vi "Configure Crop New.vi"(6 "Codec":string, 7 "State In":T1, 8 "error in (no error)":errorcluster, 9 "Time Crop Method":T3, 10 "Annotation List":T2[](array[typedef]) {"Frame Start" min=0}, 11 "Frame Grabber Data In":T4={"Camera Session"="", "Frame"=refnum, "AVI Refnum"=refnum, "Codecs"=[], "Frame number"=0, "Tracking File Refnum"=refnum, "Tick Count"=0, "Probe Object"=refnum, "Playback Probe Data"=[], "Rigid Body"={"Position"={"x (mm)"=0.0, "y (mm)"=0.0, "z (mm)"=0.0}, "Orientation"={"Pitch (rad)"=0.0, "Yaw (rad)"=0.0, "Roll (rad)"=0.0}, "Quaternion"={"qx"=0.0, "qy"=0.0, "qz"=0.0, "qw"=0.0}, "Tracked?"=FALSE}, "Total no frames playback"=0, "Video FPS"=0.0, "Camera connected?"=FALSE, "Scene"=refnum, "Cropped Frame"=refnum, "Tracker FPS"=0.0, "Crop ROI"=[], "Presentation Values"=[], "Elapsed time (ms)"=0, "Camera frames playback"=0, "Refnums"={"Live Refnum"=refnum, "Record Refnum"=refnum, "Playback Refnum"=refnum, "Frame Slider Refnum"=refnum, "Pause Refnum"=refnum, "Home Refnum"=refnum, "Set Crop Refnum"=refnum, "Clear Crop Refnum"=refnum, "stop refnum"=refnum, "Playback Rate Refnum"=refnum, "Presentation Refnum"=refnum, "Crop Time Frame Slider Refnum"=refnum, "Cancel Save Refnum"=refnum, "Reverse Playback Refnum"=refnum, "Recording Settings Refnum"=refnum, "Continuous Playback Refnum"=refnum, "Annotation Refnum"=refnum, "Export All Refnum"=refnum, "Export List Refnum"=refnum, "Fill List Refnum"=refnum, "Save Crop Refnum"=refnum, "Skip Forward Refnum"=refnum, "Skip Backward Refnum"=refnum, "Single Annotation Refnum"=refnum, "Load Refnum"=refnum, "Set Start Refnum"=refnum, "Set End Refnum"=refnum, "Add to List Refnum"=refnum, "List of Annotations Refnum"=refnum, "Camera Frame Refnum"=refnum}, "Dimensions"={"Probe Dimensions"={"Probe Width"=0.0, "Probe Depth"=1.0, "Probe Height"=0.0}, "Room Dimensions"={"Room Width"=0.0, "Room Depth"=0.0, "Room Height"=0.0}}, "Playback Data As Strings"=[], "Cropped Tracking File Refnum"=refnum, "Cropped AVI Refnum"=refnum, "Header"=[], "Total euclidian distance"=0.0, "Annotation File Path"=path "", "Playback File Path"=path "", "Size per frame"=0.0, "Ground Truth File Refnum"=refnum, "Annotation Array"=[], "Annotation TIFFs Folder"=path "", "overwriting open file?"=FALSE}) -> (0 "error out":errorcluster, 1 "Valid crop region?":bool, 2 "Saving?":bool, 3 "Frame Grabber Data Out":T4={"Camera Session"="", "Frame"=refnum, "AVI Refnum"=refnum, "Codecs"=[], "Frame number"=0, "Tracking File Refnum"=refnum, "Tick Count"=0, "Probe Object"=refnum, "Playback Probe Data"=[], "Rigid Body"={"Position"={"x (mm)"=0.0, "y (mm)"=0.0, "z (mm)"=0.0}, "Orientation"={"Pitch (rad)"=0.0, "Yaw (rad)"=0.0, "Roll (rad)"=0.0}, "Quaternion"={"qx"=0.0, "qy"=0.0, "qz"=0.0, "qw"=0.0}, "Tracked?"=FALSE}, "Total no frames playback"=0, "Video FPS"=0.0, "Camera connected?"=FALSE, "Scene"=refnum, "Cropped Frame"=refnum, "Tracker FPS"=0.0, "Crop ROI"=[], "Presentation Values"=[], "Elapsed time (ms)"=0, "Camera frames playback"=0, "Refnums"={"Live Refnum"=refnum, "Record Refnum"=refnum, "Playback Refnum"=refnum, "Frame Slider Refnum"=refnum, "Pause Refnum"=refnum, "Home Refnum"=refnum, "Set Crop Refnum"=refnum, "Clear Crop Refnum"=refnum, "stop refnum"=refnum, "Playback Rate Refnum"=refnum, "Presentation Refnum"=refnum, "Crop Time Frame Slider Refnum"=refnum, "Cancel Save Refnum"=refnum, "Reverse Playback Refnum"=refnum, "Recording Settings Refnum"=refnum, "Continuous Playback Refnum"=refnum, "Annotation Refnum"=refnum, "Export All Refnum"=refnum, "Export List Refnum"=refnum, "Fill List Refnum"=refnum, "Save Crop Refnum"=refnum, "Skip Forward Refnum"=refnum, "Skip Backward Refnum"=refnum, "Single Annotation Refnum"=refnum, "Load Refnum"=refnum, "Set Start Refnum"=refnum, "Set End Refnum"=refnum, "Add to List Refnum"=refnum, "List of Annotations Refnum"=refnum, "Camera Frame Refnum"=refnum}, "Dimensions"={"Probe Dimensions"={"Probe Width"=0.0, "Probe Depth"=1.0, "Probe Height"=0.0}, "Room Dimensions"={"Room Width"=0.0, "Room Depth"=0.0, "Room Height"=0.0}}, "Playback Data As Strings"=[], "Cropped Tracking File Refnum"=refnum, "Cropped AVI Refnum"=refnum, "Header"=[], "Total euclidian distance"=0.0, "Annotation File Path"=path "", "Playback File Path"=path "", "Size per frame"=0.0, "Ground Truth File Refnum"=refnum, "Annotation Array"=[], "Annotation TIFFs Folder"=path "", "overwriting open file?"=FALSE}, 5 "State Out":T1=enum."Multi-Crop")   [LabVIEW 2017]
uses:
  Controls/Frame Grabber Data.ctl
  <vilib>/userdefined/High Color/IMAQdx.ctl
  <vilib>/vision/Image Controls.llb/IMAQ Image.ctl
  <vilib>/vision/Avi.llb/IMAQ AVI2 Refnum.ctl
  Controls/Rigid Body Info.ctl
  Controls/Position.ctl
  Controls/Orientation.ctl
  Controls/Refnums.ctl
  Controls/Recording Settings.ctl
  Controls/Operator Settings.ctl
  Controls/Operator.ctl
  Controls/Patient Settings.ctl
  Controls/Dimensions.ctl
  Controls/Room Dimensions.ctl
  Controls/Time Crop Method.ctl
  Controls/Annotation Sequence Details.ctl
  Controls/Crop Video State.ctl
panel:
  out "Playback File Path":path
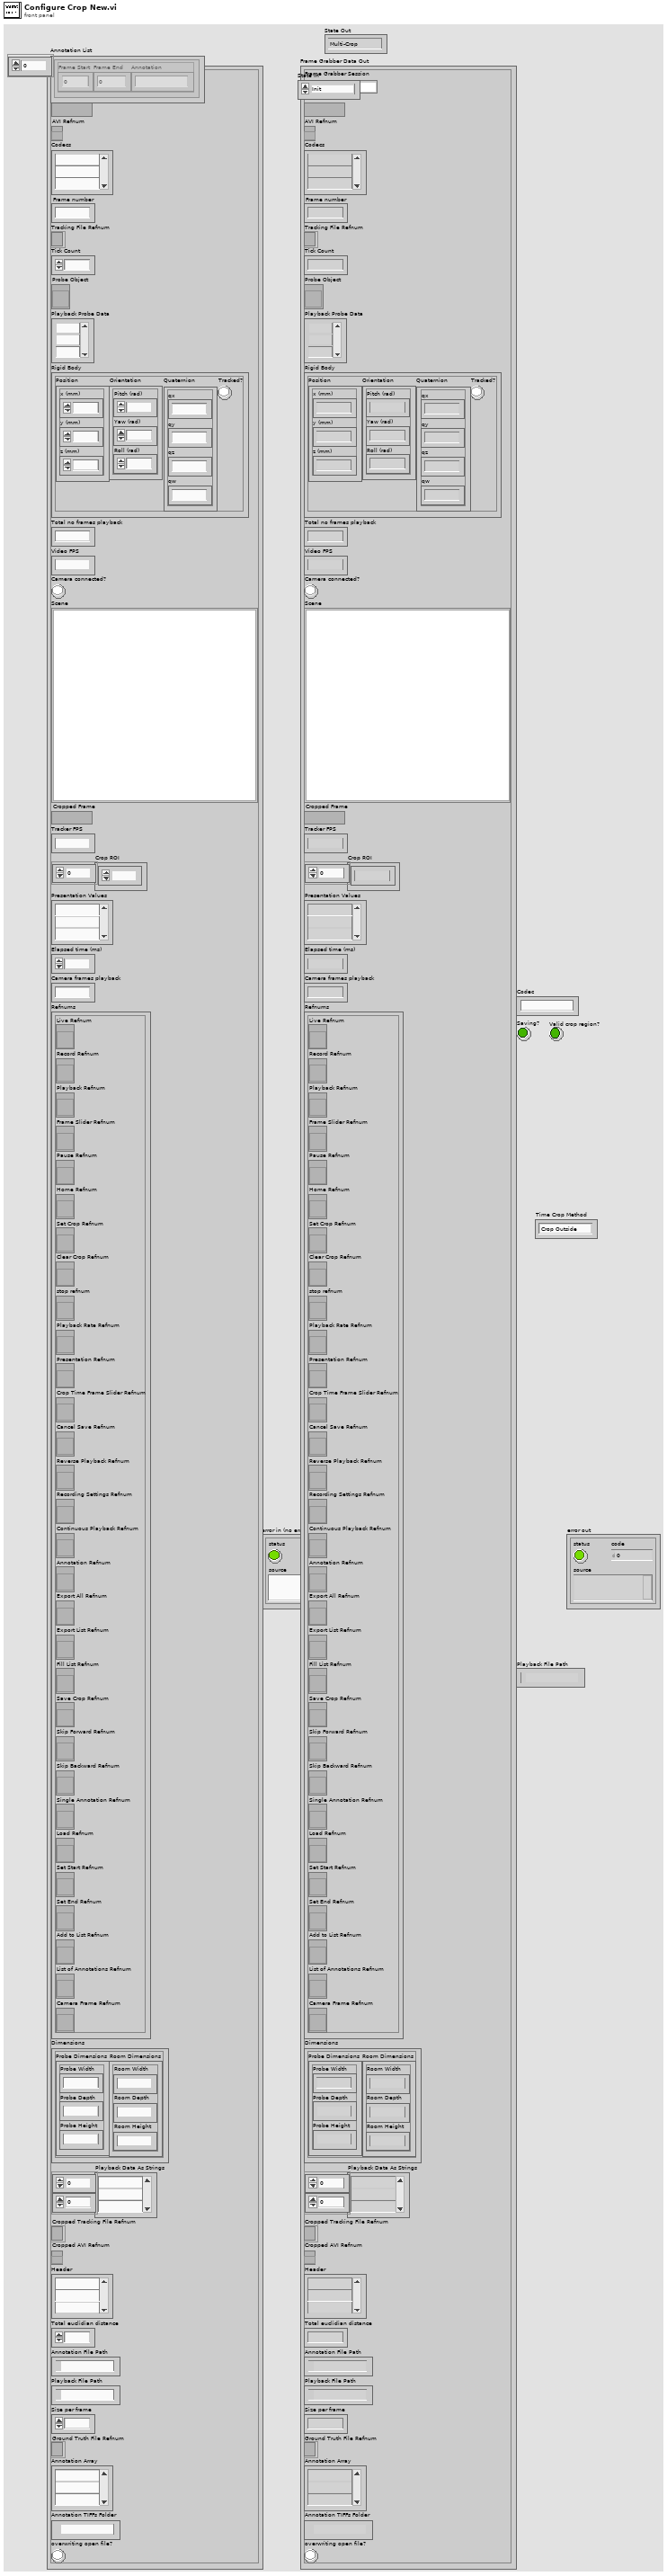
[diagram p1: front panel]
types:
  T1 = typedef "Crop Video State.ctl" = enum16{"Init", "Wait", "Load", "Playback Frame", "Save", "Export List", "Export All", "Close", "Set Crop Area", "Reset Crop Area", "Crop Inside", "Crop Outside", "Multi-Crop", "Re-Open Files", "Annotate Frame", "Annotate Clip", "Add to List", "Fill List", "Set Start", "Set End", "Error Handling", "Shutdown"}
  T2 = typedef "Annotation Sequence Details.ctl" = cluster{"Frame Start":i32, "Frame End":i32, "Annotation":string}
  T3 = typedef "Time Crop Method.ctl" = enum16{"Crop Outside", "Crop Inside"}
  T4 = typedef "Frame Grabber Data.ctl" = cluster{"Camera Session":T5, "Frame":T6, "AVI Refnum":T7, "Codecs":string[], "Frame number":u32, "Tracking File Refnum":refnum<file>, "Tick Count":u32, "Probe Object":refnum<vi>, "Playback Probe Data":dbl[][], "Rigid Body":T8, "Total no frames playback":i32, "Video FPS":dbl, "Camera connected?":bool, "Scene":refnum<vi>, "Cropped Frame":T6, "Tracker FPS":dbl, "Crop ROI":i32[], "Presentation Values":string[], "Elapsed time (ms)":u32, "Camera frames playback":u32, "Refnums":T11, "Dimensions":T12, "Playback Data As Strings":string[][], "Cropped Tracking File Refnum":refnum<file>, "Cropped AVI Refnum":T7, "Header":string[], "Total euclidian distance":dbl, "Annotation File Path":path, "Playback File Path":path, "Size per frame":dbl, "Ground Truth File Refnum":refnum<file>, "Annotation Array":string[], "Annotation TIFFs Folder":path, "overwriting open file?":bool}
  T5 = typedef "IMAQdx.ctl" = refnum<k21>
  T6 = typedef "IMAQ Image.ctl" = refnum<image>
  T7 = typedef "IMAQ AVI2 Refnum.ctl" = refnum<k20>
  T8 = typedef "Rigid Body Info.ctl" = cluster{"Position":T9, "Orientation":T10, "Quaternion":cluster{"qx":sgl, "qy":sgl, "qz":sgl, "qw":sgl}, "Tracked?":bool}
  T9 = typedef "Position.ctl" = cluster{"x (mm)":sgl, "y (mm)":sgl, "z (mm)":sgl}
  T10 = typedef "Orientation.ctl" = cluster{"Pitch (rad)":sgl, "Yaw (rad)":sgl, "Roll (rad)":sgl}
  T11 = typedef "Refnums.ctl" = cluster{"Live Refnum":refnum<vi>, "Record Refnum":refnum<vi>, "Playback Refnum":refnum<vi>, "Frame Slider Refnum":refnum<vi>, "Pause Refnum":refnum<vi>, "Home Refnum":refnum<vi>, "Set Crop Refnum":refnum<vi>, "Clear Crop Refnum":refnum<vi>, "stop refnum":refnum<vi>, "Playback Rate Refnum":refnum<vi>, "Presentation Refnum":refnum<vi>, "Crop Time Frame Slider Refnum":refnum<vi>, "Cancel Save Refnum":refnum<vi>, "Reverse Playback Refnum":refnum<vi>, "Recording Settings Refnum":refnum<vi>, "Continuous Playback Refnum":refnum<vi>, "Annotation Refnum":refnum<vi>, "Export All Refnum":refnum<vi>, "Export List Refnum":refnum<vi>, "Fill List Refnum":refnum<vi>, "Save Crop Refnum":refnum<vi>, "Skip Forward Refnum":refnum<vi>, "Skip Backward Refnum":refnum<vi>, "Single Annotation Refnum":refnum<vi>, "Load Refnum":refnum<vi>, "Set Start Refnum":refnum<vi>, "Set End Refnum":refnum<vi>, "Add to List Refnum":refnum<vi>, "List of Annotations Refnum":refnum<vi>, "Camera Frame Refnum":refnum<vi>}
  T12 = typedef "Dimensions.ctl" = cluster{"Probe Dimensions":cluster{"Probe Width":sgl, "Probe Depth":sgl, "Probe Height":sgl}, "Room Dimensions":T13}
  T13 = typedef "Room Dimensions.ctl" = cluster{"Room Width":dbl, "Room Depth":dbl, "Room Height":dbl}
  T14 = enum16{"open", "replace", "create", "open or create", "replace or create", "replace or create with confirmation"}
  T15 = cluster{"Width":u32, "Height":u32, "Frames Per Second":u32, "Codec":string, "Has Data":bool}
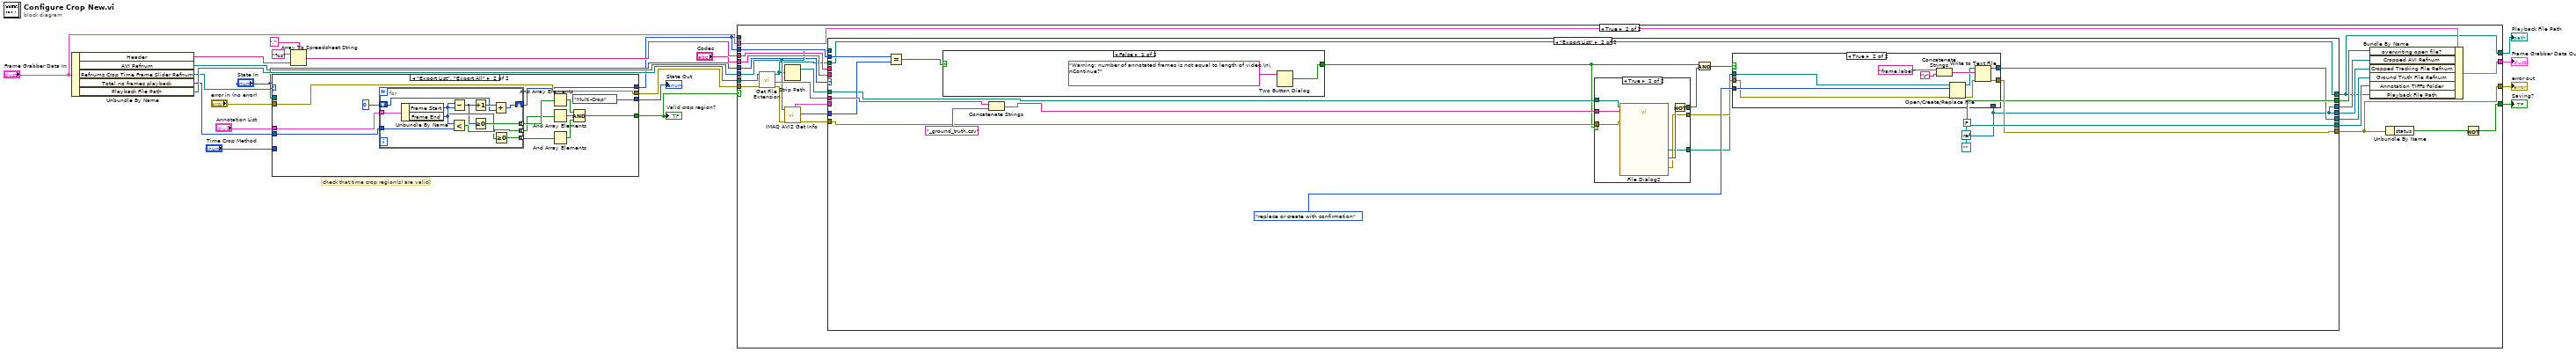
[diagram p0: block diagram]
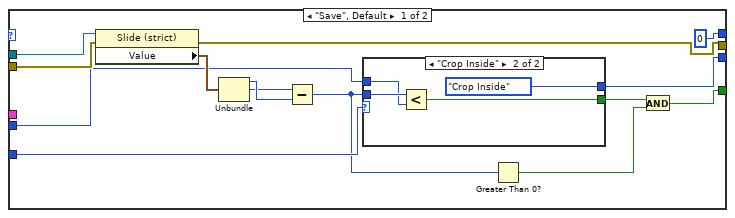
[diagram p2: hidden frame]
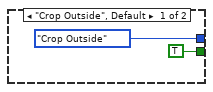
[diagram p3: hidden frame]
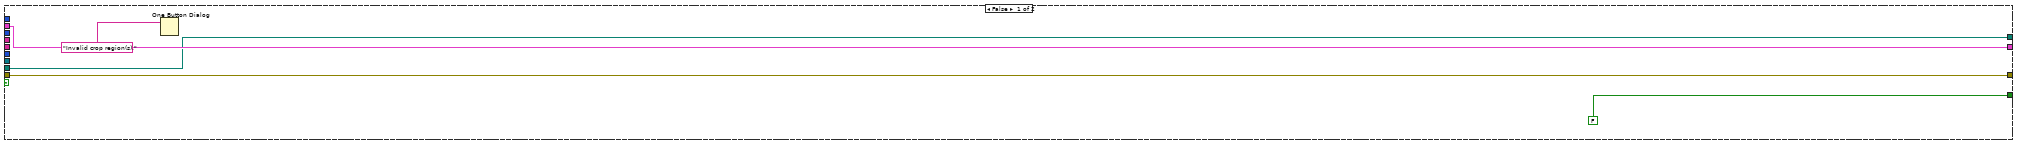
[diagram p4: hidden frame]
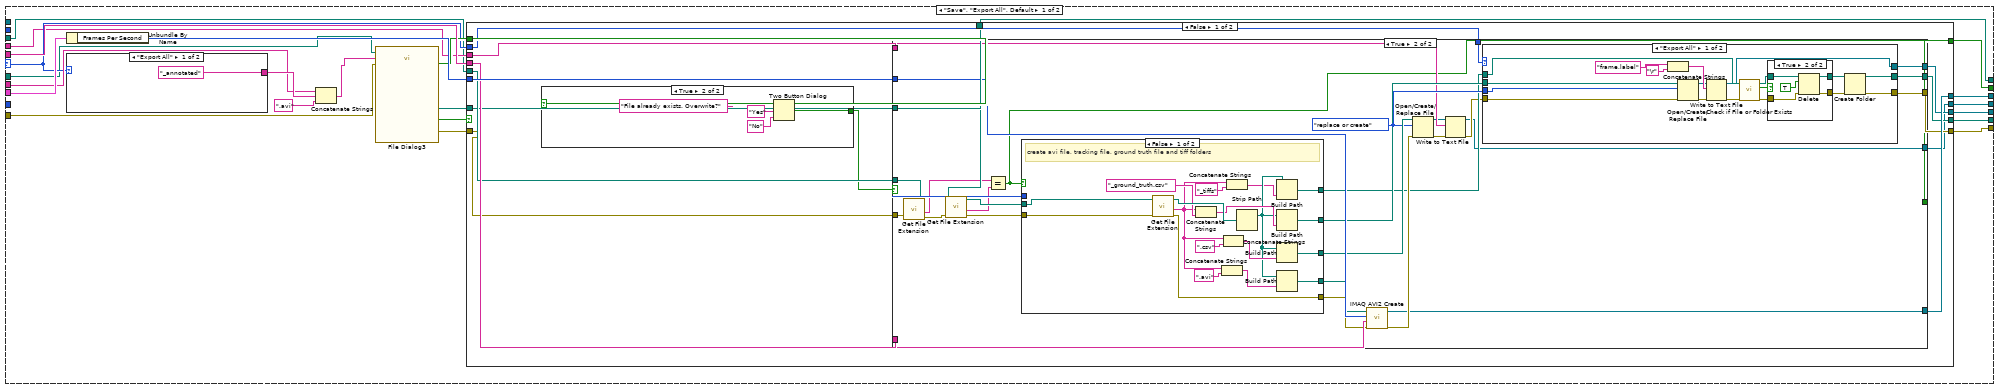
[diagram p5: hidden frame]
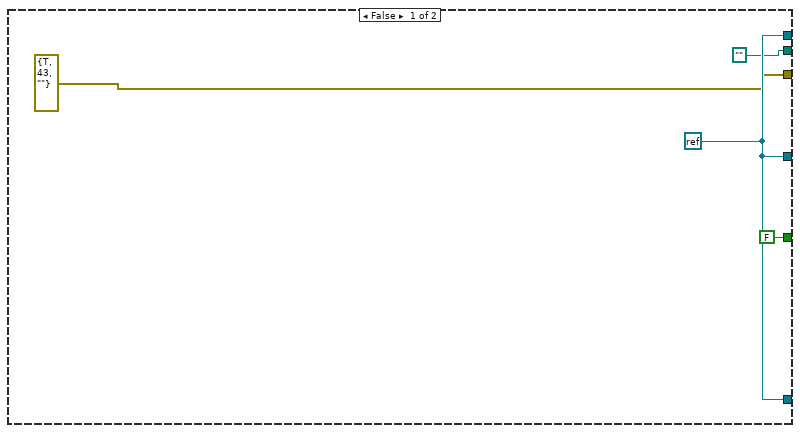
[diagram p6: hidden frame]
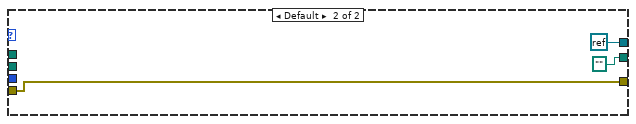
[diagram p8: hidden frame]
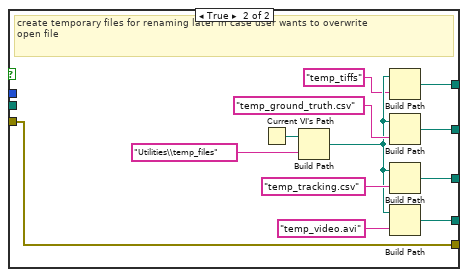
[diagram p9: hidden frame]
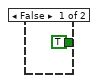
[diagram p10: hidden frame]
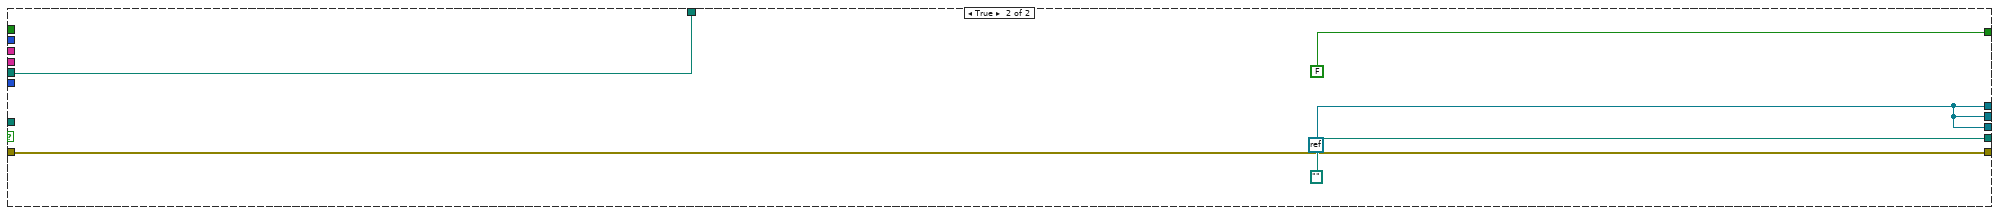
[diagram p11: hidden frame]
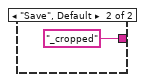
[diagram p12: hidden frame]
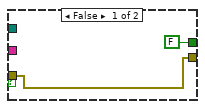
[diagram p13: hidden frame]
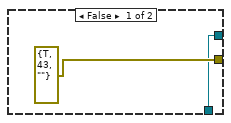
[diagram p14: hidden frame]
diagram:
  # "check that time crop region(s) are valid!"
  n1 = Unbundle By Name("Frame Grabber Data In") -> ("Header"=w16:string[], "AVI Refnum"=w3:T7, "Refnums.Crop Time Frame Slider Refnum"=w13:refnum<vi>, "Total no frames playback"=w9:i32, "Playback File Path"=w17:path)
  n2 = case shown="\"Export List\", \"Export All\"" "State In" {
    tunnel: "Annotation List" -> [_ w55]
    tunnel: w13 -> [w33 _]
    tunnel: "error in (no error)" -> [w32 w53]
    tunnel: [w31 w53] -> w11
    tunnel: "Time Crop Method" -> [w30 _]
    tunnel: w9 -> [w29 w51]
    tunnel: [w25 w46] -> w8
    tunnel: [w24 Crop_Video_State."Multi-Crop" ("State")] -> w7
    tunnel: [0 w43] -> w2
    frame "Save", Default {
      n3 = property class="Slide (strict)"(reference=w33, error in=w32) -> (error out=w31:errorcluster, "Value"=w36:cluster{i32, i32, i32})  [unwired: 1 out]
      n4 = Unbundle(w36) -> (w35:i32, w34:i32)  [unwired: 1 out]
      n5 = Subtract(x=w34, y=w35) -> (x-y=w28:i32)
      n6 = case shown="\"Crop Inside\"" w30 {
        tunnel: w28 -> [_ w41]
        tunnel: w29 -> [_ w40]
        tunnel: [TRUE w42] -> w26
        tunnel: [Crop_Video_State."Crop Outside" ("State") Crop_Video_State."Crop Inside" ("State")] -> w24
        frame "Crop Outside", Default {
        }
        frame "Crop Inside" {
          n7 = Less?(x=w41, y=w40) -> (x < y?=w42:bool)
        }
      }
      n8 = Greater Than 0?(x=w28) -> (x > 0?=w27:bool)
      n9 = And(x=w26, y=w27) -> (x .and. y?=w25:bool)
    }
    frame "Export List", "Export All" {
      n10 = for {
        tunnel: w55 -> [w66] mode=indexing
        tunnel: [w65] -> w54 mode=indexing
        tunnel: [w63] -> w52 mode=indexing
        tunnel: w51 -> [w62]
        tunnel: [w60] -> w49 mode=indexing
        shift-right: [w57] -> w43
        shift-left: 0 -> [w56]
        n11 = Unbundle By Name(w66) -> ("Frame Start"=w61:i32, "Frame End"=w64:i32)
        n12 = Less?(x=w64, y=w62) -> (x < y?=w63:bool)
        n13 = Subtract(x=w64, y=w61) -> (x-y=w59:i32)
        n14 = Increment(x=w59) -> (x+1=w58:i32)
        n15 = Greater Or Equal To 0?(x=w59) -> (x >= 0?=w65:bool)
        n16 = Add(x=w58, y=w56) -> (x+y=w57:i32)
        n17 = Greater Or Equal To 0?(x=w61) -> (x >= 0?=w60:bool)
      }
      n18 = And Array Elements(Boolean array=w54) -> (logical AND=w47:bool)
      n19 = And Array Elements(Boolean array=w52) -> (logical AND=w48:bool)
      n20 = And Array Elements(Boolean array=w49) -> (logical AND=w50:bool)
      n21 = Compound Arithmetic op=AND(w47, w48, w50) -> (w46:bool)
    }
  }
  "Valid crop region?" <- w8
  "State Out" <- w7
  n22 = Array To Spreadsheet String(delimiter (Tab)=",", array=w16, 3:"%s" ("format string")) -> (spreadsheet string=w22:string)
  n23 = case shown="True" w8 {
    tunnel: w22 -> [_ w79]
    tunnel: "Frame Grabber Data In" -> [w70 w96]
    tunnel: [w70 w95] -> w20
    tunnel: w11 -> [w69 w93]
    tunnel: w17 -> [w67 w85]
    tunnel: [FALSE ("status") w94] -> w19
    tunnel: "Codec" -> [_ w84]
    tunnel: "State In" -> [_ w73]
    tunnel: [w69 w75] -> w5
    tunnel: w2 -> [_ _]
    tunnel: w3 -> [_ w74]
    tunnel: w2 -> [_ w92]
    tunnel: [w67 w77] -> w1
    frame False {
      n24 = One Button Dialog(message="Invalid crop region(s).") -> ()  [unwired: 1 in, 1 out]
    }
    frame True {
      n25 = call <vilib>:"Get File Extension.vi"("error in (no error)"=w93, "file"=w85) -> ("error out"=w90:errorcluster, "filename without extension"=w91:string, "dup file"=w72:path)  [unwired: 5 in, 2 out]
      n26 = Strip Path(path=w72) -> (stripped path=w86:path)  [unwired: 1 out]
      n27 = call "IMAQ AVI2 Get Info"("error in (no error)"=w90, "AVI Refnum"=w74) -> ("error out"=w89:errorcluster, "Number of Frames"=w87:u32, "Frame Data"=w88:T15)  [unwired: 5 in, 2 out]
      n28 = case shown="\"Export List\"" w73 {
        selector: w73 -> [w108 _]
        tunnel: w74 -> [_ _]
        tunnel: w92 -> [_ w255]
        tunnel: w89 -> [w115 w250]
        tunnel: w91 -> [w116 w249]
        tunnel: w87 -> [_ w247]
        tunnel: w88 -> [w119 _]
        tunnel: w86 -> [w99 w241]
        tunnel: w72 -> [w98 w244]
        tunnel: w84 -> [w113 _]
        tunnel: [w109 w238] -> w83
        tunnel: [w104 w238] -> w82
        tunnel: [w107 w245] -> w75
        tunnel: [w106 path ""] -> w81
        tunnel: [w105 w239] -> w80
        tunnel: w79 -> [w103 _]
        tunnel: [w97 w244] -> w77
        tunnel: [w102 FALSE] -> w78
        frame "Save", "Export All", Default {
          n29 = Unbundle By Name(w119) -> ("Frames Per Second"=w114:u32)
          n30 = case shown="\"Export All\"" w108 {
            tunnel: ["_annotated" ("f") "_cropped" ("string")] -> w117
            frame "Export All" {
            }
            frame "Save", Default {
            }
          }
          n31 = Concatenate Strings(w116, w117, ".avi" ("string")) -> (w100:string)
          n32 = call "File Dialog3"("start path"=w99, "default name"=w100, "error in"=w115) -> ("selected path"=w111:path, "exists"=w112:bool, "cancelled"=w101:bool, "error out"=w110:errorcluster)  [unwired: 9 in]
          n33 = case shown="False" w101 {
            tunnel: w114 -> [w134 _]
            tunnel: w113 -> [w133 _]
            tunnel: w112 -> [w132 _]
            tunnel: w111 -> [w121 _]
            tunnel: w110 -> [w122 w233]
            tunnel: [w131 w232] -> w109
            tunnel: w108 -> [w130 _]
            tunnel: [w129 w233] -> w107
            tunnel: [w128 path ""] -> w106
            tunnel: [w127 w232] -> w105
            tunnel: [w126 w232] -> w104
            tunnel: w103 -> [w125 _]
            tunnel: w98 -> [w123 w230]
            tunnel: [w124 FALSE] -> w102
            tunnel: [w121 w230] -> w97
            frame False {
              n34 = case shown="True" w132 {
                tunnel: [TRUE ("T button?") w226] -> w120
                frame False {
                }
                frame True {
                  n35 = Two Button Dialog(message="File already exists. Overwrite?", 1:"No" ("F button name (\"Cancel\")"), 2:"Yes" ("T button name (\"OK\")")) -> (T button?=w226:bool)
                }
              }
              n36 = case shown="True" w120 {
                tunnel: w134 -> [_ w166]
                tunnel: w133 -> [_ w165]
                tunnel: [w138 w161] -> w131
                tunnel: w130 -> [_ w160]
                tunnel: [errorcluster {"status"=TRUE, "code"=43, "source"=""} ("error in (no error)") w157] -> w129
                tunnel: [path "" w156] -> w128
                tunnel: [w138 w155] -> w127
                tunnel: [w138 w139] -> w126
                tunnel: w125 -> [_ w152]
                tunnel: [FALSE w150] -> w124
                tunnel: w123 -> [_ w148]
                tunnel: w122 -> [_ w147]
                tunnel: w121 -> [_ w144]
                frame False {
                  w138 = refnum<k0> refnum
                }
                frame True {
                  w159 = T14."replace or create" ("operation (0:open)")
                  n37 = call <vilib>:"Get File Extension.vi"("error in (no error)"=w147, "file"=w148) -> ("error out"=w146:errorcluster, "filename without extension"=w142:string)  [unwired: 5 in, 3 out]
                  n38 = call <vilib>:"Get File Extension.vi"("error in (no error)"=w146, "file"=w144) -> ("error out"=w145:errorcluster, "filename without extension"=w141:string, "dup file"=w143:path)  [unwired: 5 in, 2 out]
                  n39 = Equal?(x=w142, y=w141) -> (x = y?=w150:bool)
                  n40 = case shown="False" w150 {
                    tunnel: w166 -> [_ _]
                    tunnel: w145 -> [w212 w216]
                    tunnel: w143 -> [w211 _]
                    tunnel: [w204 w219] -> w164
                    tunnel: [w207 w218] -> w163
                    tunnel: [w201 w217] -> w158
                    tunnel: [w196 w213] -> w154
                    tunnel: [w195 w216] -> w151
                    frame False {
                      # "create avi file, tracking file, ground truth file and tiff folders"
                      n41 = call <vilib>:"Get File Extension.vi"("error in (no error)"=w212, "file"=w211) -> ("error out"=w195:errorcluster, "filename without extension"=w199:string, "dup file"=w209:path)  [unwired: 5 in, 2 out]
                      n42 = Concatenate Strings(w199, "_ground_truth.csv" ("string")) -> (w202:string)
                      n43 = Concatenate Strings(w199, ".avi" ("string")) -> (w205:string)
                      n44 = Concatenate Strings(w199, ".csv" ("string")) -> (w208:string)
                      n45 = Concatenate Strings(w199, "_tiffs" ("string")) -> (w197:string)
                      n46 = Strip Path(path=w209) -> (stripped path=w200:path)  [unwired: 1 out]
                      n47 = Build Path(base path=w200, name or relative path=w197) -> (appended path=w196:path)
                      n48 = Build Path(base path=w200, name or relative path=w202) -> (appended path=w201:path)
                      n49 = Build Path(base path=w200, name or relative path=w208) -> (appended path=w207:path)
                      n50 = Build Path(base path=w200, name or relative path=w205) -> (appended path=w204:path)
                    }
                    frame True {
                      # "create temporary files for renaming later in case user wants to overwrite\nopen file"
                      n51 = Current VI's Path() -> (path=w224:path)
                      n52 = Build Path(base path=w224, name or relative path="Utilities\\temp_files") -> (appended path=w215:path)
                      n53 = Build Path(base path=w215, name or relative path="temp_tiffs") -> (appended path=w213:path)
                      n54 = Build Path(base path=w215, name or relative path="temp_ground_truth.csv") -> (appended path=w217:path)
                      n55 = Build Path(base path=w215, name or relative path="temp_tracking.csv") -> (appended path=w218:path)
                      n56 = Build Path(base path=w215, name or relative path="temp_video.avi") -> (appended path=w219:path)
                    }
                  }
                  n57 = call "IMAQ AVI2 Create"("error in (no error)"=w151, "Codec"=w165, "Frames Per Second"=w166, "AVI Path"=w164) -> ("error out"=w162:errorcluster, "AVI Refnum"=w161:T7)  [unwired: 6 in]
                  n58 = Open/Create/Replace File(file path (use dialog)=w163, error in=w162, operation (0:open)=w159) -> (refnum out=w140:refnum<file>, error out=w153:errorcluster)  [unwired: 3 in, 1 out]
                  n59 = Write to Text File(file (use dialog)=w140, text=w152, error in=w153) -> (refnum out=w139:refnum<file>, error out=w149:errorcluster)  [unwired: 1 in, 1 out]
                  n60 = case shown="\"Export All\"" w160 {
                    tunnel: w149 -> [w184 w192]
                    tunnel: w159 -> [w183 _]
                    tunnel: w158 -> [w182 _]
                    tunnel: [w180 w192] -> w157
                    tunnel: [w179 path ""] -> w156
                    tunnel: [w167 refnum<k0> refnum] -> w155
                    tunnel: w154 -> [w176 _]
                    frame "Export All" {
                      n61 = Concatenate Strings("frame,label" ("text"), "\r") -> (w173:string)
                      n62 = Open/Create/Replace File(file path (use dialog)=w182, error in=w184, operation (0:open)=w183) -> (refnum out=w168:refnum<file>, error out=w170:errorcluster)  [unwired: 3 in, 1 out]
                      n63 = Write to Text File(file (use dialog)=w168, text=w173, error in=w170) -> (refnum out=w167:refnum<file>, error out=w169:errorcluster)  [unwired: 1 in, 1 out]
                      n64 = call <vilib>:"Check if File or Folder Exists.vi"("error in (no error)"=w169, "path"=w176) -> ("error out"=w178:errorcluster, "file or folder exists?"=w175:bool, "dup path"=w174:path)  [unwired: 7 in]
                      n65 = case shown="True" w175 {
                        tunnel: w178 -> [w186 w191]
                        tunnel: [w186 w189] -> w181
                        tunnel: [w185 w188] -> w177
                        tunnel: w174 -> [w185 w187]
                        frame False {
                        }
                        frame True {
                          n66 = Delete(path (use dialog)=w187, entire hierarchy (F)=TRUE, error in=w191) -> (deleted path=w188:path, error out=w189:errorcluster)  [unwired: 2 in, 1 out]
                        }
                      }
                      n67 = Create Folder(path (use dialog)=w177, error in=w181) -> (created path=w179:path, error out=w180:errorcluster)  [unwired: 1 in, 1 out]
                    }
                    frame Default {
                    }
                  }
                }
              }
            }
            frame True {
              w232 = refnum<k0> refnum
            }
          }
        }
        frame "Export List" {
          w238 = refnum<k0> refnum
          n68 = Equal?(x=w255, y=w247) -> (x = y?=w254:bool)
          n69 = case shown="False" w254 {
            selector: w254 -> [_ w280]
            tunnel: [w278 w280] -> w237
            frame False {
              n70 = Two Button Dialog(message="Warning: number of annotated frames is not equal to length of video.\n\nContinue?") -> (T button?=w278:bool)  [unwired: 2 in]
            }
            frame True {
            }
          }
          n71 = Concatenate Strings(w249, "_ground_truth.csv" ("string")) -> (w240:string)
          n72 = case shown="True" w237 {
            tunnel: [FALSE w264] -> w252
            tunnel: w250 -> [w258 w263]
            tunnel: [w258 w262] -> w248
            tunnel: [_ w261] -> w243
            tunnel: w241 -> [_ w260]
            tunnel: w240 -> [_ w259]
            frame False {
            }
            frame True {
              n73 = call "File Dialog2"("start path"=w260, "default name"=w259, "error in"=w263) -> ("selected path"=w261:path, "cancelled"=w265:bool, "error out"=w262:errorcluster)  [unwired: 9 in, 1 out]
              n74 = Not(x=w265) -> (.not. x?=w264:bool)
            }
          }
          n75 = And(x=w237, y=w252) -> (x .and. y?=w251:bool)
          n76 = case shown="True" w251 {
            tunnel: T14."replace or create with confirmation" ("operation (0:open)") -> [_ w277]
            tunnel: w243 -> [_ w276]
            tunnel: w248 -> [_ w270]
            tunnel: [errorcluster {"status"=TRUE, "code"=43, "source"=""} ("error in (no error)") w269] -> w245
            tunnel: [w266 w268] -> w239
            tunnel: w238 -> [w266 _]
            frame False {
            }
            frame True {
              n77 = Concatenate Strings("frame,label" ("text"), "\r") -> (w272:string)
              n78 = Open/Create/Replace File(file path (use dialog)=w276, error in=w270, operation (0:open)=w277) -> (refnum out=w271:refnum<file>, error out=w275:errorcluster)  [unwired: 3 in, 1 out]
              n79 = Write to Text File(file (use dialog)=w271, text=w272, error in=w275) -> (refnum out=w268:refnum<file>, error out=w269:errorcluster)  [unwired: 1 in, 1 out]
            }
          }
        }
      }
      n80 = Bundle By Name(cluster=w96, "overwriting open file?"=w78, "Cropped AVI Refnum"=w83, "Cropped Tracking File Refnum"=w82, "Ground Truth File Refnum"=w80, "Annotation TIFFs Folder"=w81, "Playback File Path"=w77) -> (w95:T4)
      n81 = Unbundle By Name(w75) -> ("status"=w76:bool)
      n82 = Not(x=w76) -> (.not. x?=w94:bool)
    }
  }
  "Frame Grabber Data Out" <- w20
  "Saving?" <- w19
  "error out" <- w5
  "Playback File Path" <- w1
